vi "CRYData View Init.vi"   [LabVIEW 2013]
uses:
  Control/CRYGraph Event.ctl
  Control/CRYGraphView Property.ctl
  Control/CRYGraph Property.ctl
  Control/CRYDrag Graph.ctl
  CRYData View Global.vi
types:
  T1 = typedef "CRYDrag Graph.ctl" = cluster{"GraphType":string, "GraphData":variant}
  T2 = typedef "CRYGraphView Property.ctl" = cluster{"Queue Name":string, "Graph Proterty Array":T3[]}
  T3 = typedef "CRYGraph Property.ctl" = cluster{"LegendShow":bool, "Legend Splitter Position":dbl, "Data Names":string[], "Item Symbols":i32[], "Color Array":u32[], "Flattened Plot Property":string, "CursorShow":bool, "Flattened Cursor Property":string, "Graph Number":i32, "Flattened Scale Property":string, "PreviewShow":bool, "MagnitudeShow":bool, "PaletteShow":bool, "XYShow":bool, "FrequencyShow":bool, "Frequency Splitter Position":dbl, "XYGraph Splitter Position":dbl, "Frequency Symbols":i32[], "LegendVScrollShow":bool, "FrequencyVScrollShow":bool, "PhaseShow":bool, "Title Name":string}
  T4 = typedef "CRYGraph Event.ctl" = cluster{"EvenName":string, "TitleName":string, "GraphName":string, "GraphType":string, "Data":variant, "Queue Name":string, "DataView Number":i32}
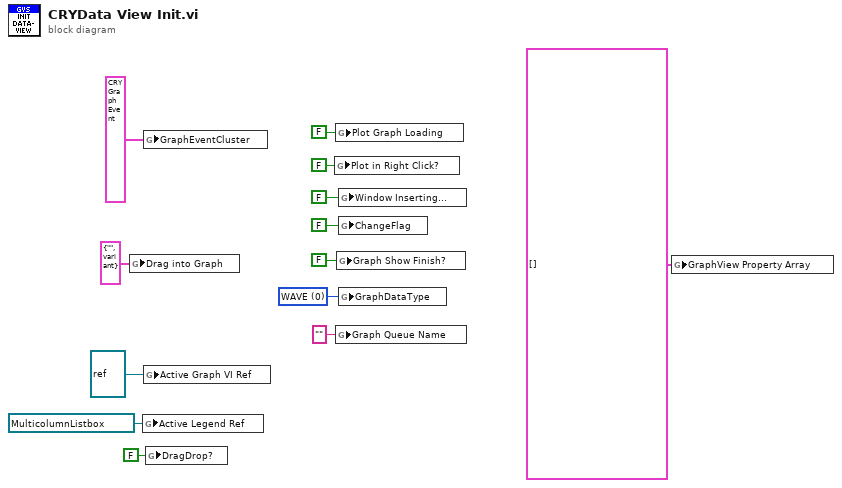
[diagram p0: block diagram]
diagram:
  w12 = u16 0 items=["WAVE", "BAR1", "POLRA", "DIGITAL", "XY ", "BAR2", "EMPTY"] ("GraphDataType")
  n1 = global write "CRYData View Global.vi" "Drag into Graph"(T1 {"GraphType"="", "GraphData"=variant} ("Drag into Graph")) -> ()
  n2 = global write "CRYData View Global.vi" "Active Legend Ref"(refnum<vi> refnum ("Active Legend Ref")) -> ()
  n3 = global write "CRYData View Global.vi" "GraphEventCluster"(T4 {"EvenName"="", "TitleName"="", "GraphName"="", "GraphType"="", "Data"=variant, "Queue Name"="", "DataView Number"=0} ("GraphEventCluster")) -> ()
  n4 = global write "CRYData View Global.vi" "Active Graph VI Ref"(refnum<vi> refnum ("Active Graph VI Ref")) -> ()
  n5 = global write "CRYData View Global.vi" "DragDrop?"(FALSE ("DragDrop?")) -> ()
  n6 = global write "CRYData View Global.vi" "Plot in Right Click?"(FALSE ("Plot in Right Click?")) -> ()
  n7 = global write "CRYData View Global.vi" "Plot Graph Loading"(FALSE ("Plot Graph Loading")) -> ()
  n8 = global write "CRYData View Global.vi" "Graph Queue Name"("" ("Graph Queue Name")) -> ()
  n9 = global write "CRYData View Global.vi" "Graph Show Finish?"(FALSE ("Graph Show Finish?")) -> ()
  n10 = global write "CRYData View Global.vi" "Window Inserting..."(FALSE ("Window Inserting...")) -> ()
  n11 = global write "CRYData View Global.vi" "ChangeFlag"(FALSE ("ChangeFlag")) -> ()
  n12 = global write "CRYData View Global.vi" "GraphDataType"(w12) -> ()
  n13 = global write "CRYData View Global.vi" "GraphView Property Array"(T2[] [] ("GraphView Property Array")) -> ()
